vi "DIs.vi"() -> ()   [LabVIEW 2019]
panel:
  in  "millisecond multiple":u32
  in  "stop":bool
  out "Output":bool
  in  "Input":bool
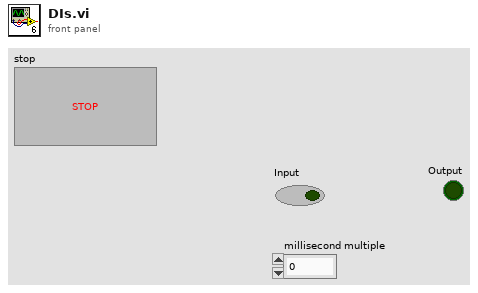
[diagram p1: front panel]
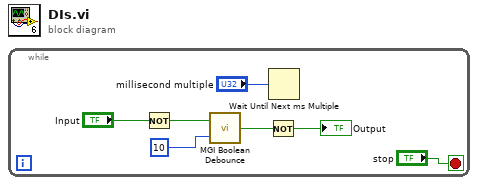
[diagram p0: block diagram]
diagram:
  n1 = while {
    stop <- "stop" stop-if-true
    n2 = Not(x="Input") -> (.not. x?=w2:bool)
    n3 = call <userlib>:"MGI Boolean Debounce.vi"("Filter Length"=10, "Input"=w2) -> ("Output"=w6:bool)
    n4 = Not(x=w6) -> (.not. x?=→"Output":bool)
    n5 = Wait Until Next ms Multiple(millisecond multiple="millisecond multiple") -> ()  [unwired: 1 out]
  }
